vi "Large File Write.vi"(5 "Username":string, 6 "Password":string, 7 "Address":string, 8 "Error In":errorcluster) -> (0 "Error Out":errorcluster)   [LabVIEW 2018, in "Tests.lvlib" / "SFTP File.lvlib"]
uses:
  SFTP File.lvlib
  src/Toolkit/API/SFTP File/API/Typedefs/Flags.ctl
  src/Toolkit/API/Typedefs/Permissions.ctl
  src/Toolkit/API/Typedefs/Modes.ctl
  src/Toolkit/API/SFTP Attributes/SFTP Attributes.lvclass/SFTP Attributes.ctl
  src/Toolkit/API/SSH/SSH.lvclass/SSH.ctl
  src/Toolkit/API/SSH/Utility/Read Shared Library.vi
  src/Toolkit/API/SFTP Attributes/Support/Create from SFTP File.vi
  src/Toolkit/Support/Check Status.vi
  src/Toolkit/API/SFTP Attributes/Support/Destroy to SFTP File.vi
  src/Toolkit/API/SFTP File/SFTP File.lvclass
  src/Toolkit/Toolkit.lvlib
  src/Toolkit/API/SFTP Attributes/SFTP Attributes.lvclass
  <vilib>/addons/_JKI Toolkits/Caraya/classes/Test/Test.lvclass
  <vilib>/addons/_JKI Toolkits/Caraya/classes/Assert/Assert.lvclass
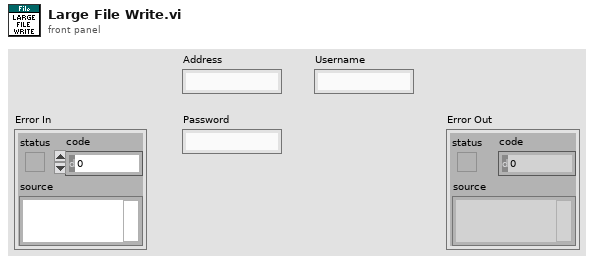
[diagram p1: front panel]
types:
  T1 = enum16{"open", "replace", "create", "open or create", "replace or create", "replace or create with confirmation"}
  T2 = typedef "Toolkit.lvlib/Permissions.ctl" = cluster{"Owner":T3, "Group":T3, "Others":T3}
  T3 = typedef "Toolkit.lvlib/Modes.ctl" = cluster{"Read":bool, "Write":bool, "Execute":bool}
  T4 = typedef "Toolkit.lvlib/SFTP File.lvclass/Flags.ctl" = cluster{"Read":bool, "Write":bool, "Append":bool, "Create":bool, "Truncate":bool, "Exclude":bool}
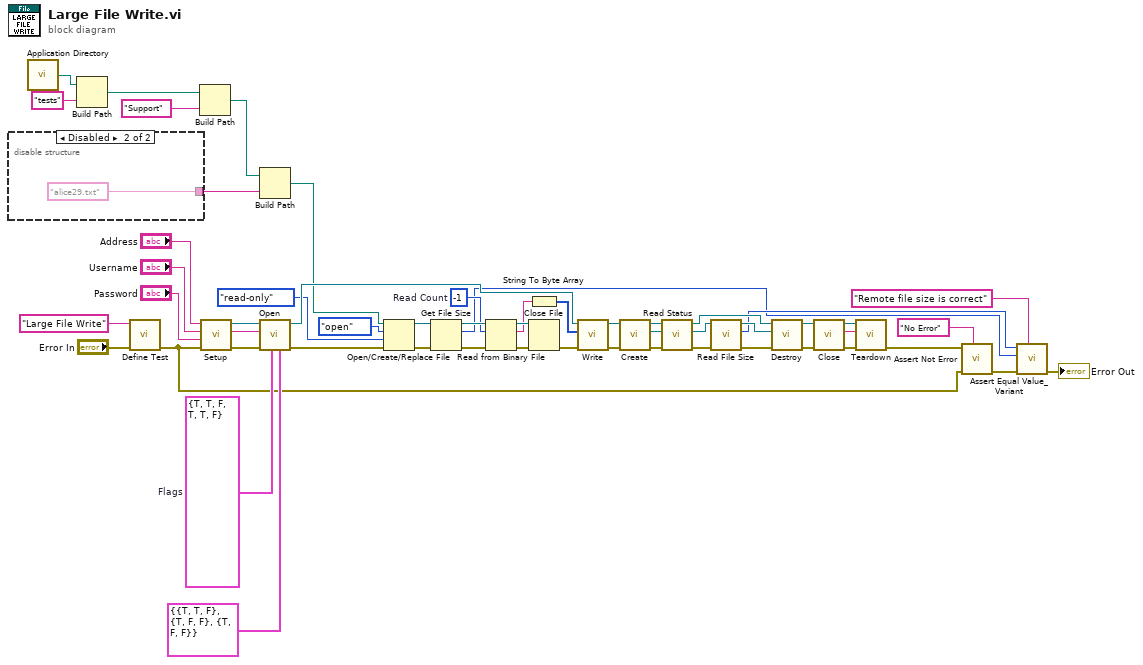
[diagram p0: block diagram]
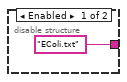
[diagram p2: hidden frame]
diagram:
  w29 = -1  # Read Count
  w49 = T4 {"Read"=TRUE, "Write"=TRUE, "Append"=FALSE, "Create"=TRUE, "Truncate"=TRUE, "Exclude"=FALSE}  # Flags
  n1 = disable-structure "Diagram Disable Structure" shown="Disabled" {
    disable-tunnel: ["EColi.txt" ("name or relative path") "alice29.txt" ("name or relative path")] -> w13
    frame Enabled {
    }
    frame Disabled {
    }
  }
  n2 = call <vilib>:"Application Directory.vi"() -> ("Application Directory"=w36:path)
  n3 = Build Path(base path=w36, name or relative path="tests") -> (appended path=w34:path)
  n4 = call <vilib>:"Define Test.vi"("error in (no error)"="Error In", "Label (VI Title)"="Large File Write") -> ("error out"=w7:errorcluster)  [unwired: 9 in]
  n5 = Build Path(base path=w34, name or relative path="Support") -> (appended path=w32:path)
  n6 = call "Setup.vi"("Error In"=w7, "Password"="Password", "Username"="Username", "Address"="Address") -> ("Error Out"=w48:errorcluster, "Temporary File"=w37:string, "SFTP"=w51:refnum<class "SFTP.lvclass">)  [unwired: 5 in]
  n7 = Build Path(base path=w32, name or relative path=w13) -> (appended path=w31:path)
  n8 = call "Open.vi"("Permissions"=T2 {"Owner"={"Read"=TRUE, "Write"=TRUE, "Execute"=FALSE}, "Group"={"Read"=TRUE, "Write"=FALSE, "Execute"=FALSE}, "Others"={"Read"=TRUE, "Write"=FALSE, "Execute"=FALSE}}, "Flags"=w49, "Error In"=w48, "Remote Path"=w37, "SFTP"=w51) -> ("Error Out"=w43:errorcluster, "SFTP File"=w50:refnum<class "SFTP File.lvclass">)  [unwired: 5 in]
  n9 = Open/Create/Replace File(file path (use dialog)=w31, error in=w43, operation (0:open)=T1."open", access (0:read/write)=enum16{"read/write", "read-only", "write-only"}."read-only") -> (refnum out=w40:refnum<file>, error out=w38:errorcluster)  [unwired: 2 in, 1 out]
  n10 = Get File Size(file=w40, error in=w38) -> (refnum out=w39:refnum<file>, size (in bytes)=w1:i64, 0:w30:errorcluster)
  n11 = Read from Binary File(8:w30, 10:w29, 11:w39) -> (0:w25:errorcluster, 2:w27:string, 3:w28:refnum<file>)  [unwired: 3 in, 1 out]
  n12 = String To Byte Array(string=w27) -> (unsigned byte array=w26:u8[])
  n13 = Close File(refnum=w28, error in=w25) -> (error out=w24:errorcluster)  [unwired: 1 out]
  n14 = call "Write.vi"("Error In"=w24, "Data"=w26, "SFTP File In"=w50) -> ("Error Out"=w21:errorcluster, "SFTP File Out"=w23:refnum<class "SFTP File.lvclass">)  [unwired: 6 in, 1 out]
  n15 = call-poly "Create.vi"("Error In"=w21, "SFTP File In"=w23) -> ("Error Out"=w20:errorcluster, "SFTP Attributes"=w19:refnum<class "SFTP Attributes.lvclass">, "SFTP File Out"=w22:refnum<class "SFTP File.lvclass">)  [unwired: 7 in]
  n16 = call "Read Status.vi"("Error In"=w20, "Attributes In"=w19, "SFTP File In"=w22) -> ("Error Out"=w11:errorcluster, "Attributes Out"=w12:refnum<class "SFTP Attributes.lvclass">, "SFTP File Out"=w17:refnum<class "SFTP File.lvclass">)  [unwired: 6 in]
  n17 = call "Read File Size.vi"("Error In"=w11, "SFTP Attributes In"=w12) -> ("Error Out"=w18:errorcluster, "File Size"=w2:u64, "SFTP Attribute Out"=w16:refnum<class "SFTP Attributes.lvclass">)  [unwired: 7 in]
  n18 = call-poly "Destroy.vi"("Error In"=w18, "SFTP Attributes"=w16, "SFTP File In"=w17) -> ("Error Out"=w14:errorcluster, "SFTP File Out"=w15:refnum<class "SFTP File.lvclass">)  [unwired: 7 in]
  n19 = call "Close.vi"("Error In"=w14, "SFTP File"=w15) -> ("Error Out"=w45:errorcluster, "Remote Path"=w47:string, "SFTP"=w46:refnum<class "SFTP.lvclass">)  [unwired: 7 in]
  n20 = call "Teardown.vi"("Error In"=w45, "Temporary File"=w47, "SFTP"=w46) -> ("Error Out"=w8:errorcluster)  [unwired: 8 in]
  n21 = call <vilib>:"Assert Not Error.vi"("Label"="No Error", "error in (no error)"=w7, "Not Error?"=w8) -> ("error out"=w5:errorcluster)  [unwired: 8 in]
  n22 = call <vilib>:"Assert Equal Value_Variant.vi"("Label"="Remote file size is correct", "error in (no error)"=w5, "Y"=w1, "X"=w2) -> ("error out"=→"Error Out":errorcluster)  [unwired: 7 in]
